vi "set_frequency.vi"(8 "error in":errorcluster, 11 "RF Generator settings":T1) -> (0 "error out":errorcluster)   [LabVIEW 2013, in "HP8662A_RF_Generator.lvclass"]
uses:
  HP8662A_RF_Generator.lvclass
  <vilib>/Instr/_visa.llb/GPIB Status Boolean Array.ctl
  RF_Generator_settings.ctl
  GPIB.lvclass
panel:
  out "status":T2
  out "GPIB channel #":string
  out "resulting string":string
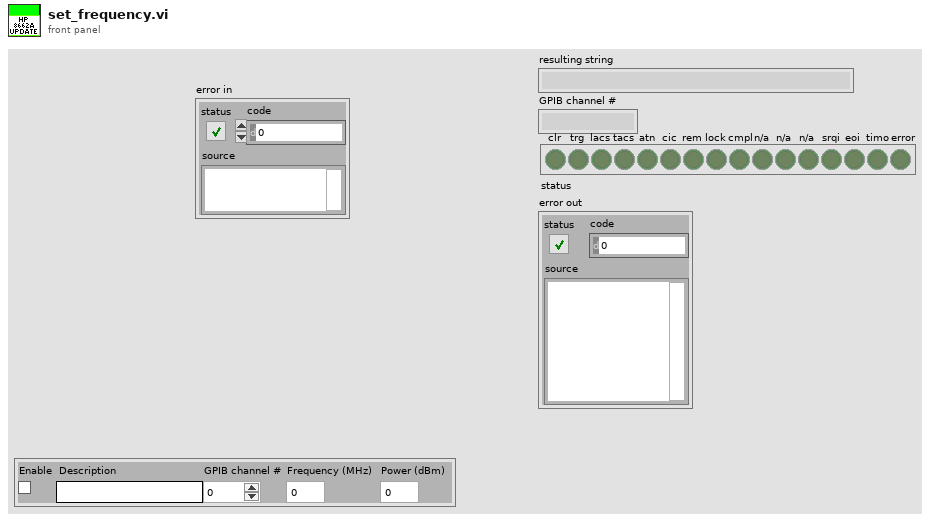
[diagram p1: front panel]
types:
  T1 = typedef "GPIB.lvclass/RF_Generator_settings.ctl" = cluster{"Enable":bool, "Description":string, "GPIB channel #":u8, "Frequency (MHz)":dbl, "Power (dBm)":dbl}
  T2 = typedef "GPIB Status Boolean Array.ctl" = bool[]
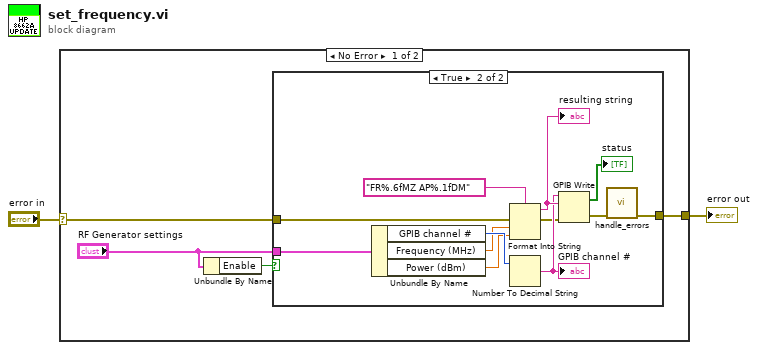
[diagram p0: block diagram]
diagram:
  n1 = case shown="No Error" "error in" {
    selector: "error in" -> [w4 w20]
    tunnel: [w3 w20] -> w1
    frame No Error {
      n2 = Unbundle By Name("RF Generator settings") -> ("Enable"=w5:bool)
      n3 = case shown="True" w5 {
        tunnel: "RF Generator settings" -> [_ w12]
        tunnel: w4 -> [w7 w10]
        tunnel: [w7 w11] -> w3
        frame False {
        }
        frame True {
          n4 = Unbundle By Name(w12) -> ("GPIB channel #"=w13:u8, "Frequency (MHz)"=w9:dbl, "Power (dBm)"=w8:dbl)
          n5 = Format Into String(format string="FR%.6fMZ AP%.1fDM", error in=w10, w9, w8) -> (resulting string=w18:string, error out=w15:errorcluster)  [unwired: 1 in]
          "resulting string" <- w18
          n6 = Number To Decimal String(number=w13) -> (decimal integer string=w17:string)  [unwired: 1 in]
          "GPIB channel #" <- w17
          n7 = GPIB Write(0:w17, 1:w18, 3:w15) -> (5:→"status":bool[], 6:w14:errorcluster)  [unwired: 2 in]
          n8 = call "handle_errors.vi"("error in (no error)"=w14) -> ("error out"=w11:errorcluster)  [unwired: 14 in]
        }
      }
    }
    frame Error {
    }
  }
  "error out" <- w1
